vi "stringToByteArray.vi"(8 "error in (no error)":errorcluster, 10 "Prepend Size":bool, 11 "String":string) -> (0 "error out":errorcluster, 3 "byte array":u8[](array[numeric]))   [LabVIEW 2013, in "BSON.lvlib"]
uses:
  BSON.lvlib
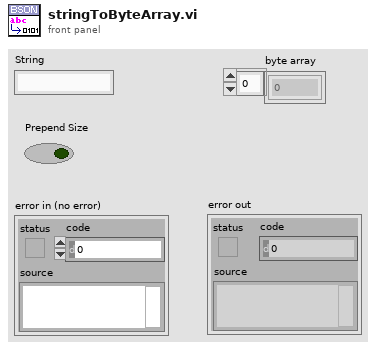
[diagram p1: front panel]
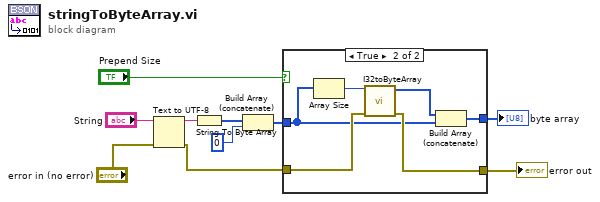
[diagram p0: block diagram]
diagram:
  n1 = Text to UTF-8(8:"error in (no error)", 11:"String") -> (0:w3:errorcluster, 3:w8:string)
  n2 = String To Byte Array(string=w8) -> (unsigned byte array=w9:u8[])
  n3 = Build Array (concatenate)(w9, u8 0) -> (w4:u8[])
  n4 = case shown="True" "Prepend Size" {
    tunnel: w4 -> [w11 w14]
    tunnel: w3 -> [w12 w17]
    tunnel: [w12 w16] -> w2
    tunnel: [w11 w13] -> w1
    frame False {
    }
    frame True {
      n5 = Array Size(array=w14) -> (size(s)=w18:i32)
      n6 = call "I32toByteArray.vi"("error in (no error)"=w17, "I32"=w18) -> ("error out"=w16:errorcluster, "LittleEndianByteArray"=w15:u8[])  [unwired: 8 in]
      n7 = Build Array (concatenate)(w15, w14) -> (w13:u8[])
    }
  }
  "error out" <- w2
  "byte array" <- w1
